vi "test_GetItemInformationFromProjects_SampleProjectWithExternalDep.vi"() -> (3 "Pass?":bool)   [LabVIEW 2019, in "Tests.SolutionBuilder.lvlib"]
uses:
  Tests.SolutionBuilder.lvlib
  SolutionBuilder/SolutionBuilder.lvclass
  SolutionBuilder/ProjectItem/ProjectItem.lvclass
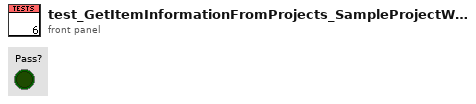
[diagram p1: front panel]
types:
  T1 = cluster{"Relative Path from 1 to 2":path, string[]}[]
  T2 = typedef "SolutionBuilder.lvlib/SolutionBuilder.lvclass/ProjectItemMap.ctl" = map{path, refnum<class "ProjectItem.lvclass">[]}
  T3 = cluster{"Relative Path from 1 to 2":path, string[]}
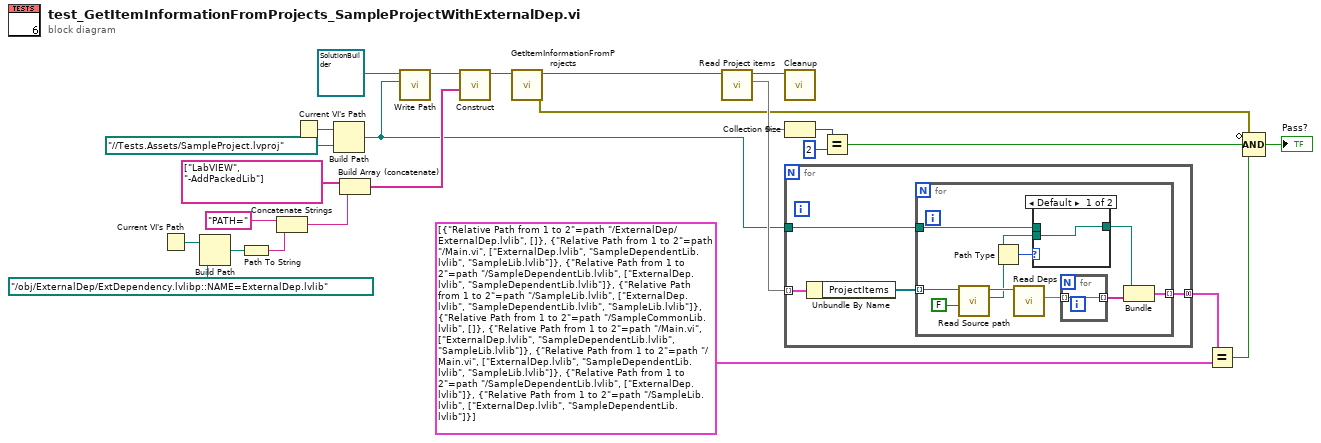
[diagram p0: block diagram]
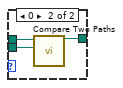
[diagram p2: hidden frame]
diagram:
  n1 = Current VI's Path() -> (path=w12:path)
  n2 = Build Path(base path=w12, name or relative path=path "../obj/ExternalDep/ExtDependency.lvlibp::NAME=ExternalDep.lvlib" ("Path")) -> (appended path=w14:path)
  n3 = Path To String(path=w14) -> (string=w6:string)
  n4 = Concatenate Strings("PATH=" ("string"), w6) -> (w4:string)
  n5 = Current VI's Path() -> (path=w24:path)
  n6 = Build Path(base path=w24, name or relative path=path "../../Tests.Assets/SampleProject.lvproj" ("Path")) -> (appended path=w7:path)
  n7 = Build Array (concatenate)(string[] ["LabVIEW", "-AddPackedLib"] ("App.Args"), w4) -> (w13:string[])
  n8 = call "Write Path.vi"("Path"=w7, "SolutionBuilder in"=refnum<class "SolutionBuilder.lvclass"> refnum) -> ("SolutionBuilder out"=w18:refnum<class "SolutionBuilder.lvclass">)  [unwired: 9 in]
  n9 = call "Construct.vi"("App.Args"=w13, "SolutionBuilder in"=w18) -> ("SolutionBuilder out"=w10:refnum<class "SolutionBuilder.lvclass">)  [unwired: 8 in, 1 out]
  n10 = call "GetItemInformationFromProjects.vi"("SolutionBuilder in"=w10) -> ("error out"=w3:errorcluster, "SolutionBuilder out"=w9:refnum<class "SolutionBuilder.lvclass">)  [unwired: 9 in]
  n11 = call "Read Project items.vi"("SolutionBuilder in"=w9) -> ("Project items"=w20:T2, "SolutionBuilder out"=w17:refnum<class "SolutionBuilder.lvclass">)  [unwired: 9 in]
  n12 = call "Cleanup.vi"("SolutionBuilder in"=w17) -> ()  [unwired: 9 in, 2 out]
  n13 = Collection Size(1:w20) -> (0:w22:i32)
  n14 = for {
    tunnel: w20 -> [w29] mode=indexing
    tunnel: [w27] -> w8 mode=concatenating
    tunnel: w7 -> [w26]
    n15 = Unbundle By Name(w29) -> ("ProjectItems"=w28:refnum<class "ProjectItem.lvclass">[])
    n16 = for {
      tunnel: w28 -> [w36] mode=indexing
      tunnel: [w37] -> w27 mode=indexing
      tunnel: w26 -> [w30]
      n17 = call "Read Source path.vi"("Force abs path? (T)"=FALSE, "ProjectItem in"=w36) -> ("Source path"=w31:path, "ProjectItem out"=w35:refnum<class "ProjectItem.lvclass">)  [unwired: 8 in]
      n18 = Path Type(1:w31) -> (0:w33:i16)
      n19 = call "Read Deps.vi"("ProjectItem in"=w35) -> ("Deps"=w39:set{string})  [unwired: 9 in, 1 out]
      n20 = case shown="Default" w33 {
        tunnel: w31 -> [w40 w41]
        tunnel: [w40 w43] -> w32
        tunnel: w30 -> [_ w42]
        frame Default {
        }
        frame 0 {
          n21 = call <vilib>:"Compare Two Paths.vi"("Path 2"=w41, "Path 1"=w42) -> ("Relative Path from 1 to 2"=w43:path)  [unwired: 6 in, 3 out]
        }
      }
      n22 = for {
        tunnel: w39 -> [w44] mode=indexing
        tunnel: [w44] -> w38 mode=indexing
      }
      n23 = Bundle("Relative Path from 1 to 2"=w32, w38) -> (w37:T3)  [unwired: 1 in]
    }
  }
  n24 = Equal?(x=w22, y=2) -> (x = y?=w19:bool)
  n25 = Equal?(x=w8, y=T1 [{"Relative Path from 1 to 2"=path "../ExternalDep/ExternalDep.lvlib", []}, {"Relative Path from 1 to 2"=path "../Main.vi", ["ExternalDep.lvlib", "SampleDependentLib.lvlib", "SampleLib.lvlib"]}, {"Relative Path from 1 to 2"=path "../SampleDependentLib.lvlib", ["ExternalDep.lvlib", "SampleDependentLib.lvlib"]}, {"Relative Path from 1 to 2"=path "../SampleLib.lvlib", ["ExternalDep.lvlib", "SampleDependentLib.lvlib", "SampleLib.lvlib"]}, {"Relative Path from 1 to 2"=path "../SampleCommonLib.lvlib", []}, {"Relative Path from 1 to 2"=path "../Main.vi", ["ExternalDep.lvlib", "SampleDependentLib.lvlib", "SampleLib.lvlib"]}, {"Relative Path from 1 to 2"=path "../Main.vi", ["ExternalDep.lvlib", "SampleDependentLib.lvlib", "SampleLib.lvlib"]}, {"Relative Path from 1 to 2"=path "../SampleDependentLib.lvlib", ["ExternalDep.lvlib"]}, {"Relative Path from 1 to 2"=path "../SampleLib.lvlib", ["ExternalDep.lvlib", "SampleDependentLib.lvlib"]}] ("Array")) -> (x = y?=w16:bool)
  n26 = Compound Arithmetic op=AND(invert w3, w19, w16) -> (→"Pass?":bool)
